vi "getDataSubset.vi"(0 "U8ArrayParserManualIndexing in":refnum<class "U8ArrayParserManualIndexing.lvclass">, 5 "Length":i32, 7 "Index":i32, 9 "OverrideSwapBytes":bool, 11 "error in (no error)":errorcluster) -> (4 "U8ArrayParserManualIndexing out":refnum<class "U8ArrayParserManualIndexing.lvclass">, 6 "Data":u8[](array[numeric]), 8 "Index out":i32, 15 "error out":errorcluster)   [LabVIEW 2016, in "RTUtilities.lvlib" / "U8ArrayParserManualIndexing.lvclass"]
uses:
  U8ArrayParserManualIndexing.lvclass
  U8ArrayParserManualIndexing.lvclass/U8ArrayParserManualIndexing.ctl
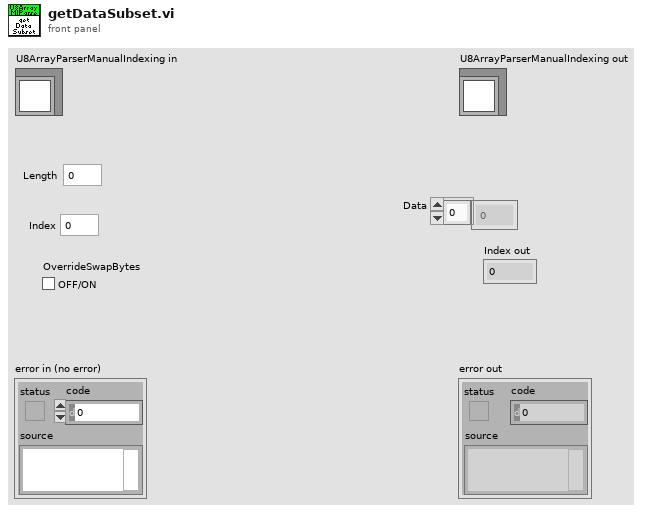
[diagram p1: front panel]
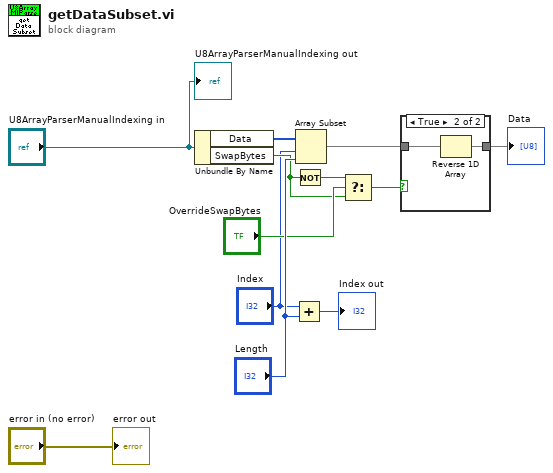
[diagram p0: block diagram]
diagram:
  n1 = Unbundle By Name("U8ArrayParserManualIndexing in") -> ("Data"=w12:u8[], "SwapBytes"=w7:bool)
  n2 = Add(x="Index", y="Length") -> (x+y=→"Index out":i32)
  n3 = Not(x=w7) -> (.not. x?=w8:bool)
  n4 = Array Subset(array=w12, index="Index", length="Length") -> (w5:u8[])
  n5 = Select(t=w8, s="OverrideSwapBytes", f=w7) -> (s? t:f=w6:bool)
  n6 = case shown="True" w6 {
    tunnel: w5 -> [w13 w15]
    tunnel: [w13 w14] -> w4
    frame False {
    }
    frame True {
      n7 = Reverse 1D Array(array=w15) -> (reversed array=w14:u8[])
    }
  }
  "Data" <- w4
  "error out" <- "error in (no error)"
  "U8ArrayParserManualIndexing out" <- "U8ArrayParserManualIndexing in"
